vi "Apply Angle.vi"(8 "error in (no error)":errorcluster, 10 "ccw servo angle (rad)":dbl, 11 "servo motor in":refnum<class "NI_Robotics_Starter Kit Servo Motor.lvclass">) -> (0 "error out":errorcluster, 3 "servo motor out":refnum<class "NI_Robotics_Starter Kit Servo Motor.lvclass">)   [LabVIEW 2017, in "NI_Robotics_Starter Kit Servo Motor.lvclass"]
uses:
  <vilib>/robotics/Starter Kit/Servo Motor/NI_Robotics_Starter Kit Servo Motor.lvclass
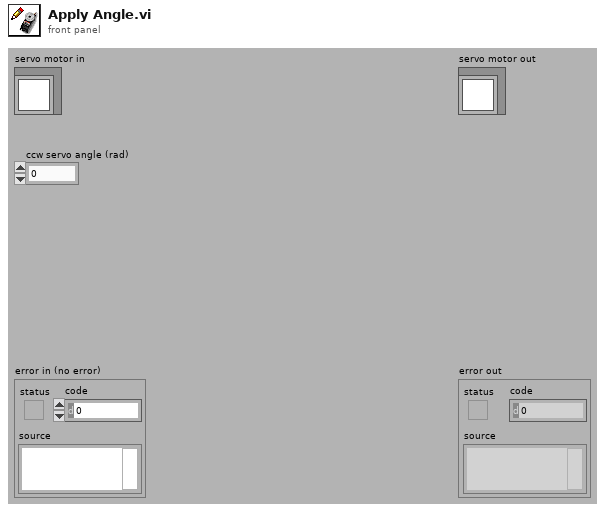
[diagram p1: front panel]
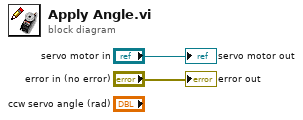
[diagram p0: block diagram]
diagram:
  "error out" <- "error in (no error)"
  "servo motor out" <- "servo motor in"
